vi "IO Channel Empty Check.vi"(1 "Enable Y Output":bool=TRUE, 2 "Enable Y Input":bool=TRUE, 3 "Enable X Output":bool=TRUE, 4 "Enable X Input":bool=TRUE) -> (0 "Required Channels Empty":bool)   [LabVIEW 2013]
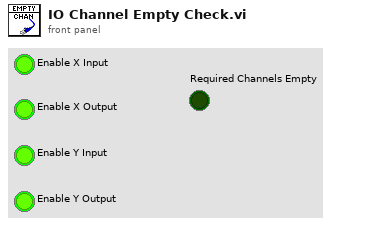
[diagram p1: front panel]
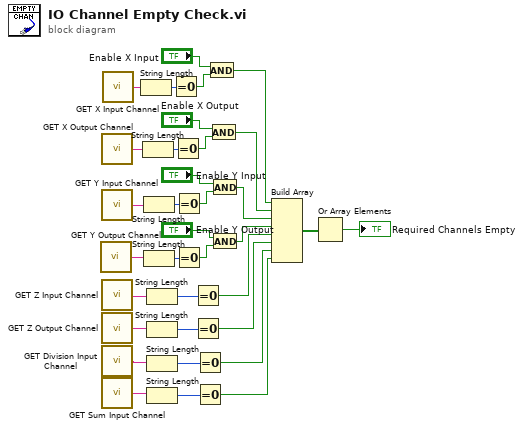
[diagram p0: block diagram]
diagram:
  n1 = call "GET Y Output Channel.vi"() -> ("Y Output Channel"=w20:string)
  n2 = call "GET X Output Channel.vi"() -> ("X Output Channel"=w28:string)
  n3 = call "GET Y Input Channel.vi"() -> ("Y Input Channel"=w24:string)
  n4 = call "GET Z Input Channel.vi"() -> ("Z Input Channel"=w5:string)
  n5 = call "GET Z Output Channel.vi"() -> ("Z Output Channel"=w4:string)
  n6 = call "GET Division Input Channel.vi"() -> ("Division Input Channel"=w3:string)
  n7 = call "GET Sum Input Channel.vi"() -> ("Sum Input Channel"=w2:string)
  n8 = call "GET X Input Channel.vi"() -> ("X Input Channel"=w34:string)
  n9 = String Length(string=w34) -> (length=w33:i32)
  n10 = String Length(string=w28) -> (length=w30:i32)
  n11 = String Length(string=w24) -> (length=w26:i32)
  n12 = String Length(string=w20) -> (length=w22:i32)
  n13 = String Length(string=w5) -> (length=w18:i32)
  n14 = String Length(string=w4) -> (length=w17:i32)
  n15 = String Length(string=w3) -> (length=w16:i32)
  n16 = String Length(string=w2) -> (length=w15:i32)
  n17 = Equal To 0?(x=w33) -> (x = 0?=w32:bool)
  n18 = Equal To 0?(x=w30) -> (x = 0?=w29:bool)
  n19 = Equal To 0?(x=w26) -> (x = 0?=w25:bool)
  n20 = Equal To 0?(x=w22) -> (x = 0?=w21:bool)
  n21 = Equal To 0?(x=w18) -> (x = 0?=w9:bool)
  n22 = Equal To 0?(x=w17) -> (x = 0?=w8:bool)
  n23 = Equal To 0?(x=w16) -> (x = 0?=w7:bool)
  n24 = Equal To 0?(x=w15) -> (x = 0?=w6:bool)
  n25 = And(x="Enable X Input", y=w32) -> (x .and. y?=w13:bool)
  n26 = And(x="Enable X Output", y=w29) -> (x .and. y?=w12:bool)
  n27 = And(x="Enable Y Input", y=w25) -> (x .and. y?=w11:bool)
  n28 = And(x="Enable Y Output", y=w21) -> (x .and. y?=w10:bool)
  n29 = Build Array(w13, w12, w11, w10, w9, w8, w7, w6) -> (w14:bool[])
  n30 = Or Array Elements(Boolean array=w14) -> (logical OR=→"Required Channels Empty":bool)
